vi "_Start.vi"(8 "error in (no error)":errorcluster, 11 "Loop Data In":T1) -> (0 "error out":errorcluster, 3 "Loop Data":T1)   [LabVIEW 2020, in "Vecto.lvlib" / "RemoteDataService.lvclass"]
uses:
  RemoteDataService.lvclass
  Loop Data.ctl
  SequenceCountService/SequenceCountService.lvclass
  Published Group.ctl
  Packet.ctl
  <vilib>/IlluminatedG/IG Protoc/LV-Proto/Message/Message.lvclass
  Subscription.ctl
  Subscription Info.ctl
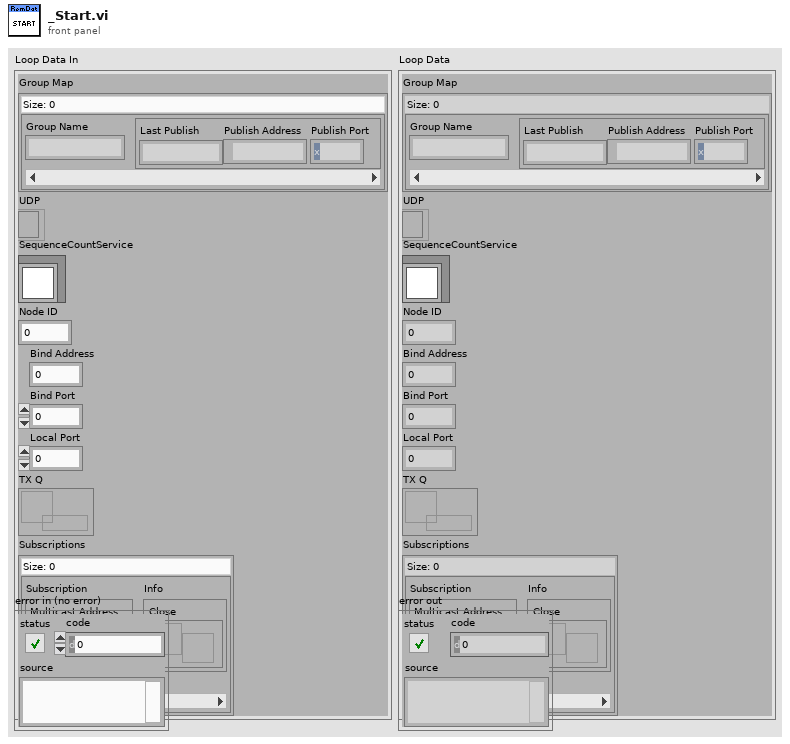
[diagram p1: front panel]
types:
  T1 = typedef "Vecto.lvlib/RemoteDataService.lvclass/Loop Data.ctl" = cluster{"Group Map":map{string, T2}, "UDP":refnum<k16>, "SequenceCountService":refnum<class "SequenceCountService.lvclass">, "Node ID":u32, "Bind Address":u32, "Bind Port":u16, "Local Port":u16, "TX Q":refnum<queue>, "Subscriptions":map{T3, T4}}
  T2 = typedef "Vecto.lvlib/RemoteDataService.lvclass/Published Group.ctl" = cluster{"Last Publish":dbl, "Publish Address":u32, "Publish Port":u16}
  T3 = typedef "Vecto.lvlib/RemoteDataService.lvclass/Subscription.ctl" = cluster{"Multicast Address":string, "Multicast Port":u16}
  T4 = typedef "Vecto.lvlib/RemoteDataService.lvclass/Subscription Info.ctl" = cluster{"Close":refnum<user-event>}
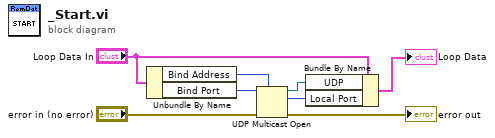
[diagram p0: block diagram]
diagram:
  n1 = Unbundle By Name("Loop Data In") -> ("Bind Address"=w8:u32, "Bind Port"=w7:u16)
  n2 = UDP Multicast Open(7:w8, 8:"error in (no error)", 11:w7) -> (0:→"error out":errorcluster, 2:w4:u16, 3:w5:refnum<k16>)  [unwired: 1 in, 1 out]
  n3 = Bundle By Name(cluster="Loop Data In", "UDP"=w5, "Local Port"=w4) -> (→"Loop Data":T1)
